vi "Log to TDMS.vi"(5 "group name in (Untitled)":string, 7 "channel name(s) in (Untitled)":string[](array[string]), 10 "Array":dbl[][](array[numeric]), 11 "TDMS File Path In":string) -> (3 "String":string)   [LabVIEW 2019]
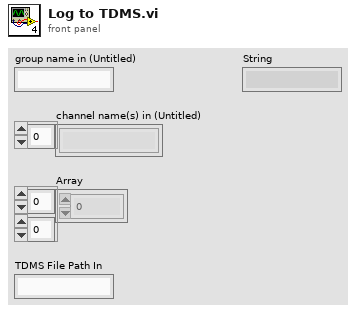
[diagram p1: front panel]
types:
  T1 = enum16{"open", "open or create", "create or replace", "create", "open (read-only)"}
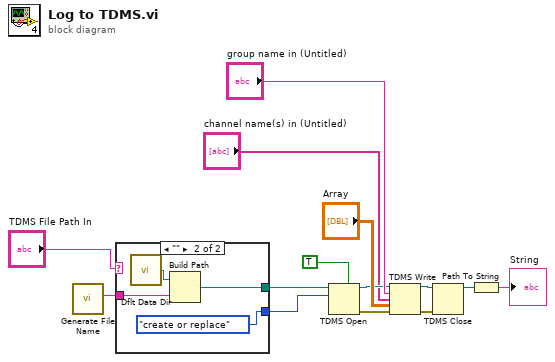
[diagram p0: block diagram]
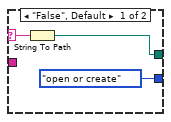
[diagram p2: hidden frame]
diagram:
  n1 = call "Generate File Name.vi"() -> ("file name"=w12:string)  [unwired: 9 in, 1 out]
  n2 = case shown="\"\"" "TDMS File Path In" {
    selector: "TDMS File Path In" -> [w16 _]
    tunnel: [T1."open or create" ("operation (0:open)") T1."create or replace" ("operation (0:open)")] -> w7
    tunnel: [w15 w19] -> w8
    tunnel: w12 -> [_ w18]
    frame "False", Default {
      n3 = String To Path(string=w16) -> (path=w15:path)
    }
    frame "" {
      n4 = call <vilib>:"Dflt Data Dir.vi"() -> ("App:Default Data Directory"=w21:path)
      n5 = Build Path(base path=w21, name or relative path=w18) -> (appended path=w19:path)
    }
  }
  n6 = TDMS Open(5:TRUE ("create index file? (T)"), 10:w7, 11:w8) -> (0:w9:errorcluster, 3:w10:refnum<k34>)  [unwired: 4 in]
  n7 = TDMS Write(0:w10, 5:"group name in (Untitled)", 7:"channel name(s) in (Untitled)", 9:"Array", 11:w9) -> (4:w1:refnum<k34>, 15:w2:errorcluster)  [unwired: 1 in, 2 out]
  n8 = TDMS Close(8:w2, 11:w1) -> (3:w4:path)  [unwired: 1 out]
  n9 = Path To String(path=w4) -> (string=→"String":string)
